vi "Set Detection.vi"(8 "error in (no error)":errorcluster, 9 "Optical Path":T1=1 items=["Eyepieces"=1, "Right"=2, "Bottom"=3, "Left"=4], 10 "Filter Position":T2=1 items=["1"=1, "2"=2, "3"=3, "4"=4, "5"=5, "6"=6], 11 "Application in":refnum<class "Application.lvclass">) -> (0 "error out":errorcluster, 3 "Application out":refnum<class "Application.lvclass">)   [LabVIEW 2018, in "Application.lvlib" / "Application.lvclass"]
uses:
  Application.lvclass
  Hardware/Ti2/ti2lv/ti2_filterPos.ctl
  Hardware/Ti2/ti2lv/ti2_lightPath.ctl
  Application.lvclass/Application.ctl
  Hardware/Virtual Microscope Messages/Set Detection Msg/Set Detection Msg.lvclass/Set Detection Msg.ctl
  <vilib>/ActorFramework/Message Enqueuer/Message Enqueuer.lvclass/Message Enqueuer.ctl
  <vilib>/ActorFramework/Message Enqueuer/Enqueue.vi
  Hardware/Virtual Microscope Messages/Set Detection Msg/Set Detection Msg.lvclass
  C:/Program Files/National Instruments/LabVIEW 2018/vi.lib/ActorFramework/Message/Message.lvclass
  <vilib>/ActorFramework/Message Priority Queue/Priority Enqueue.vi
  Hardware/Ti2/ti2lv/ti2lv.lvlib
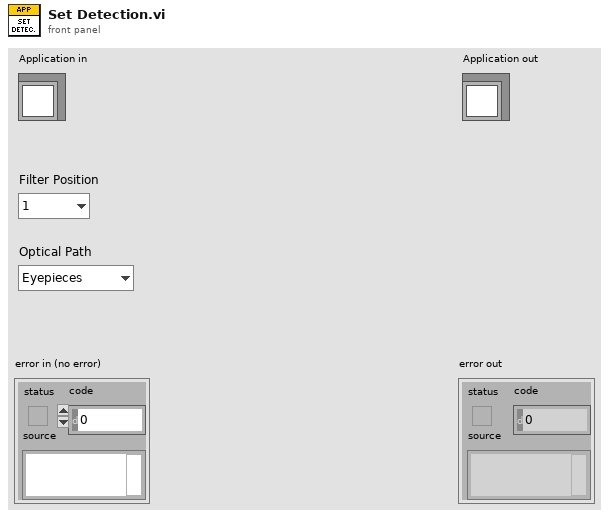
[diagram p1: front panel]
types:
  T1 = typedef "ti2lv.lvlib/ti2_lightPath.ctl" = i32
  T2 = typedef "ti2lv.lvlib/ti2_filterPos.ctl" = u16
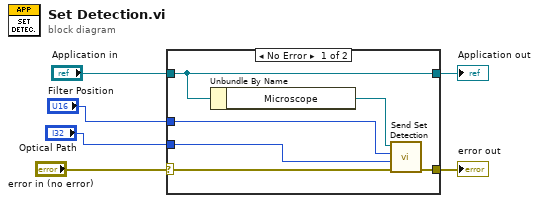
[diagram p0: block diagram]
diagram:
  n1 = case shown="No Error" "error in (no error)" {
    selector: "error in (no error)" -> [w9 w14]
    tunnel: [w10 w14] -> w5
    tunnel: [w12 w13] -> w3
    tunnel: "Application in" -> [w12 w13]
    tunnel: "Filter Position" -> [w8 _]
    tunnel: "Optical Path" -> [w7 _]
    frame No Error {
      n2 = Unbundle By Name(w12) -> ("Microscope"=w11:refnum<class "Message Enqueuer.lvclass">)
      n3 = call "Send Set Detection.vi"("error in (no error)"=w9, "Optical Path"=w7, "Filter Position"=w8, "Message Enqueuer"=w11) -> ("error out"=w10:errorcluster)  [unwired: 6 in, 1 out]
    }
    frame Error {
    }
  }
  "error out" <- w5
  "Application out" <- w3
